vi "Write to Excel waveform.vi"() -> ()   [LabVIEW 2022 SP3]
panel:
  out "error out":errorcluster
  in  "file path (use dialog)":path
  out "Waveform Graph":dbl[](graph)
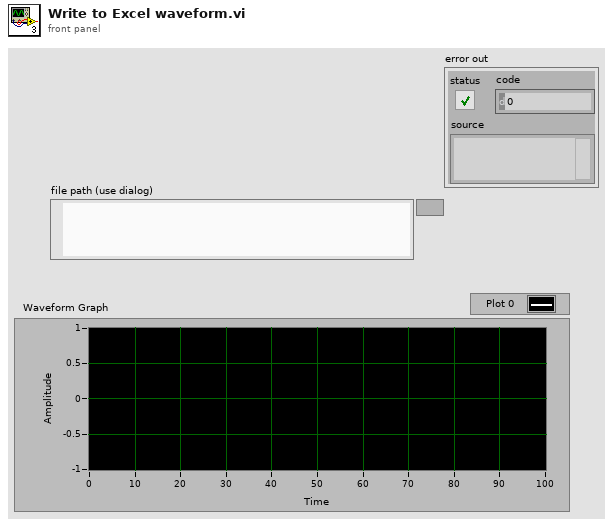
[diagram p1: front panel]
types:
  T1 = enum16{"open", "replace", "create", "open or create", "replace or create", "replace or create with confirmation"}
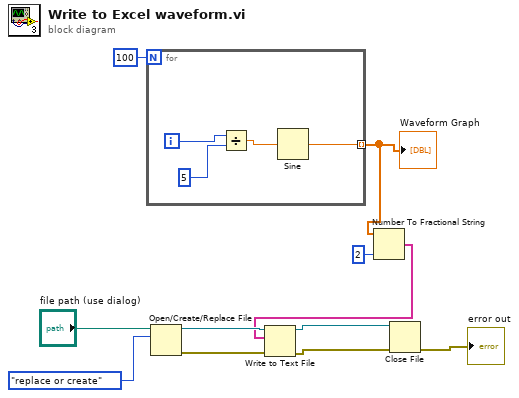
[diagram p0: block diagram]
diagram:
  n1 = for {
    N: 100 -> [_]
    tunnel: [w12] -> w2 mode=indexing
    i -> [w15]
    n2 = Divide(x=w15, y=5) -> (x/y=w13:dbl)
    n3 = Sine(x=w13) -> (sin(x)=w12:dbl)
  }
  "Waveform Graph" <- w2
  n4 = Open/Create/Replace File(file path (use dialog)="file path (use dialog)", operation (0:open)=T1."replace or create") -> (refnum out=w8:refnum<file>, error out=w7:errorcluster)  [unwired: 4 in, 1 out]
  n5 = Number To Fractional String(number=w2, precision (6)=i16 2) -> (F-format string=w1:string[])  [unwired: 2 in]
  n6 = Write to Text File(file (use dialog)=w8, text=w1, error in=w7) -> (refnum out=w6:refnum<file>, error out=w5:errorcluster)  [unwired: 1 in, 1 out]
  n7 = Close File(refnum=w6, error in=w5) -> (error out=→"error out":errorcluster)  [unwired: 1 out]
